vi "glb_Library Configuration Globals.vi"() -> ()   [LabVIEW 2012]
doc: "Some basic configuration settings. These can be set from LabVIEW or via a LuaVIEW bootstrap script."
panel:
  in  "persistence path":path=path "Local Connection"
  in  "time format":string="%Y/%m/%d %H:%M:%S%2u"
  in  "resource base path":path
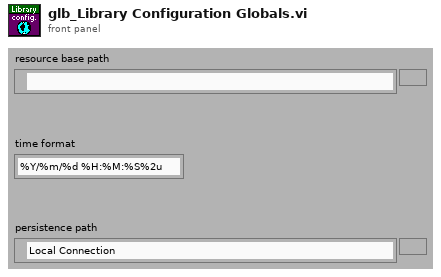
[diagram p1: front panel]
diagram:
